vi "Create Splash Screen User Event.vi"(8 "error in (no error)":errorcluster) -> (0 "error out":errorcluster, 3 "Splash Screen Event":refnum<user-event>)   [LabVIEW 2016, in "SLL Splash Screen.lvlib"]
uses:
  SLL Splash Screen.lvlib
  _Typedefs/Splash Screen Data.ctl
  _Typedefs/User Event LV2 Command.ctl
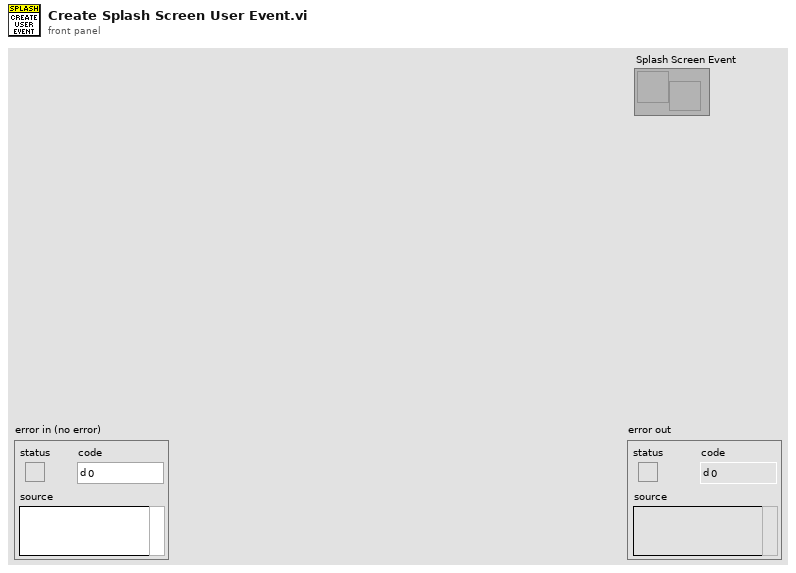
[diagram p1: front panel]
types:
  T1 = typedef "SLL Splash Screen.lvlib/User Event LV2 Command.ctl" = enum16{"Create", "Generate", "Delete"}
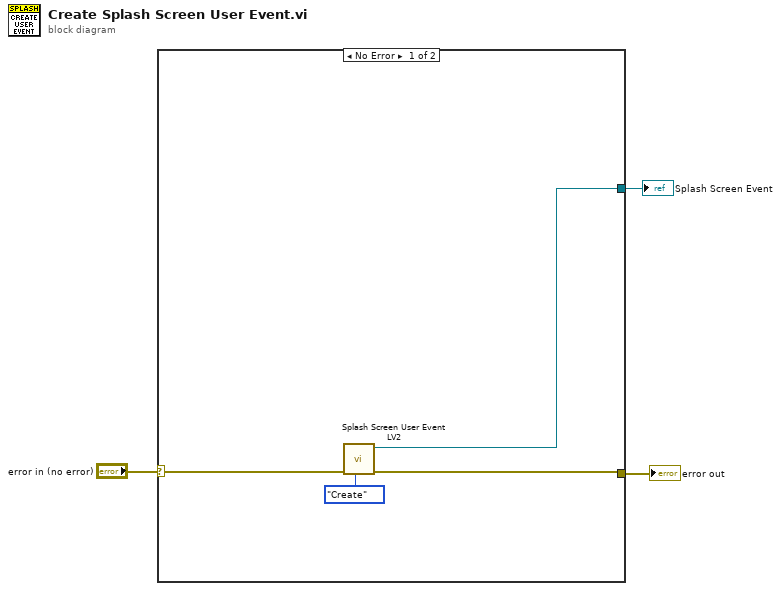
[diagram p0: block diagram]
diagram:
  n1 = case shown="No Error" "error in (no error)" {
    selector: "error in (no error)" -> [w7 w8]
    tunnel: [w6 w8] -> w2
    tunnel: [w5 _] -> w1
    frame No Error {
      n2 = call "Splash Screen User Event LV2.vi"("Command"=User_Event_LV2_Command."Create", "error in (no error)"=w7) -> ("error out"=w6:errorcluster, "Splash Screen Event"=w5:refnum<user-event>)  [unwired: 8 in]
    }
    frame Error {
    }
  }
  "error out" <- w2
  "Splash Screen Event" <- w1
